vi "Read Graph refs.vi"(8 "error in (no error)":errorcluster, 11 "MassSpectrumExtractor in":refnum<class "MassSpectrumExtractor.lvclass">) -> (0 "error out":errorcluster, 2 "Graph refs":T1, 3 "MassSpectrumExtractor out":refnum<class "MassSpectrumExtractor.lvclass">)   [LabVIEW 2014, in "MassSpectrumExtractor.lvclass"]
uses:
  MassSpectrumExtractor.lvclass
  Graph with cursors/Graph with cursors XControl.xctl
  MassSpectrumExtractor.lvclass/MassSpectrumExtractor.ctl
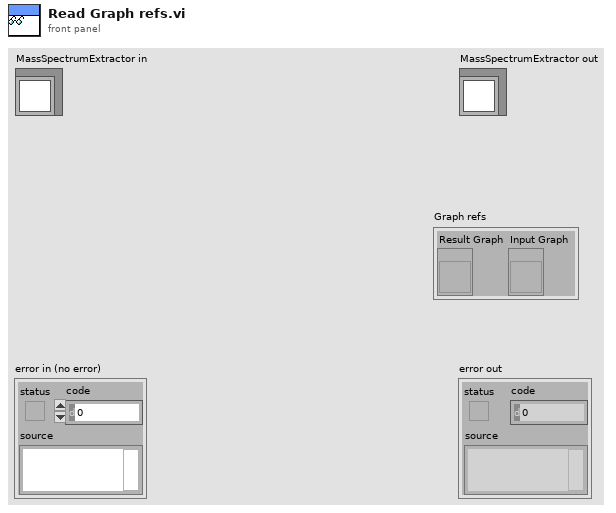
[diagram p1: front panel]
types:
  T1 = cluster{"Result Graph":refnum<vi>, "Input Graph":refnum<vi>}
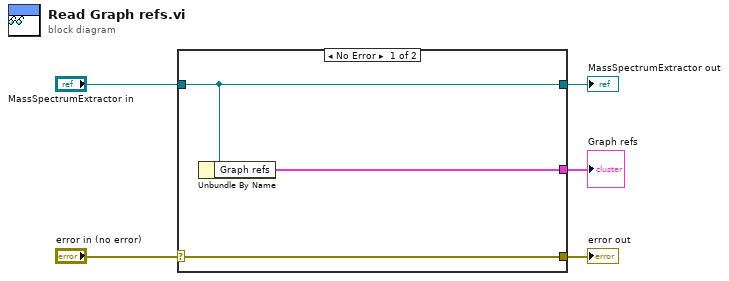
[diagram p0: block diagram]
diagram:
  n1 = case shown="No Error" "error in (no error)" {
    selector: "error in (no error)" -> [w8 w9]
    tunnel: [w8 w9] -> w4
    tunnel: [w7 w10] -> w2
    tunnel: "MassSpectrumExtractor in" -> [w7 w10]
    tunnel: [w6 _] -> w1
    frame No Error {
      n2 = Unbundle By Name(w7) -> ("Graph refs"=w6:T1)
    }
    frame Error {
    }
  }
  "error out" <- w4
  "MassSpectrumExtractor out" <- w2
  "Graph refs" <- w1
